vi "Set DC Current Ramp.vi"(0 "Address":string="24", 1 "Current":dbl format="%.3e") -> ()   [LabVIEW 2012]
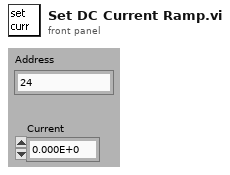
[diagram p1: front panel]
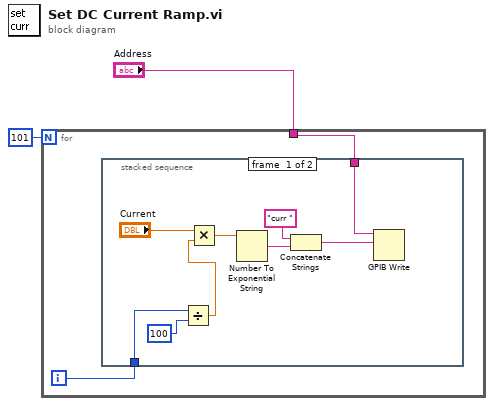
[diagram p0: block diagram]
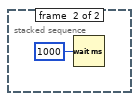
[diagram p2: hidden frame]
diagram:
  n1 = for {
    N: 101 -> [_]
    tunnel: "Address" -> [w4]
    i -> [w3]
    n2 = stacked-sequence {
      tunnel: w4 -> [w10 _]
      tunnel: w3 -> [w6 _]
      frame #0 {
        n3 = Divide(x=w6, y=100) -> (x/y=w8:dbl)
        n4 = Multiply(x="Current", y=w8) -> (x*y=w7:dbl)
        n5 = Number To Exponential String(number=w7) -> (E-format string=w12:string)  [unwired: 3 in]
        n6 = Concatenate Strings("curr " ("string"), w12) -> (w11:string)
        n7 = GPIB Write(0:w10, 1:w11) -> ()  [unwired: 3 in, 2 out]
      }
      frame #1 {
        n8 = Wait (ms)(milliseconds to wait=u32 1000) -> ()  [unwired: 1 out]
      }
    }
  }
